vi "attachBall.vi"(0 "object in":refnum<class "KickToSkill.lvclass">, 1 "Dest":dbl[](array[numeric]), 2 "robotPos":dbl[](array[numeric]), 3 "Dist":dbl, 5 "error in (no error)":errorcluster) -> (14 "object out":refnum<class "KickToSkill.lvclass">, 15 "DestArray":dbl[](array[numeric]), 19 "error out":errorcluster)   [LabVIEW 2024, in "KickToSkill.lvclass"]
uses:
  KickToSkill.lvclass
  <vilib>/Analysis/coordinate.llb/2D Cartesian Coordinate Rotation (Scalar).vi
  <vilib>/Analysis/NI_AALPro.lvlib
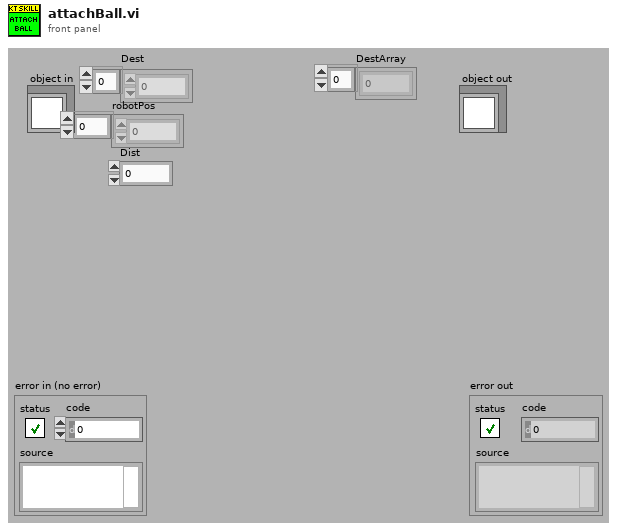
[diagram p1: front panel]
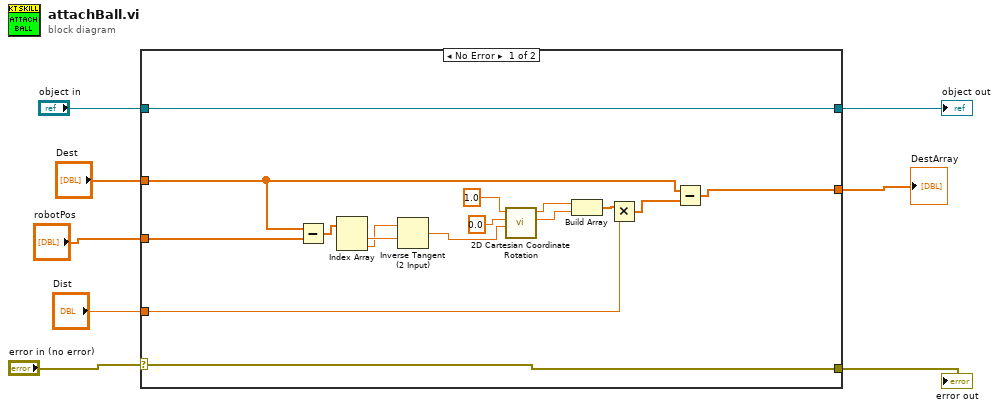
[diagram p0: block diagram]
diagram:
  n1 = case shown="No Error" "error in (no error)" {
    selector: "error in (no error)" -> [w23 w27]
    tunnel: [w23 w27] -> w7
    tunnel: [w24 w26] -> w5
    tunnel: "object in" -> [w24 w26]
    tunnel: [w15 w25] -> w4
    tunnel: "Dest" -> [w12 w25]
    tunnel: "Dist" -> [w14 _]
    tunnel: "robotPos" -> [w13 _]
    frame No Error {
      n2 = Subtract(x=w12, y=w13) -> (x-y=w11:dbl[])
      n3 = Index Array(array=w11) -> (element #1=w10:dbl, element #2=w9:dbl)  [unwired: 2 in]
      n4 = Inverse Tangent (2 Input)(1:w10, 2:w9) -> (0:w16:dbl)
      n5 = call-poly <vilib>:"2D Cartesian Coordinate Rotation.vi"("theta"=w16, "y"=0.0, "x"=1.0) -> ("y out"=w19:dbl, "x out"=w20:dbl)  [unwired: 6 in, 1 out]
      n6 = Build Array(w20, w19) -> (w18:dbl[])
      n7 = Multiply(x=w18, y=w14) -> (x*y=w17:dbl[])
      n8 = Subtract(x=w12, y=w17) -> (x-y=w15:dbl[])
    }
    frame Error {
    }
  }
  "error out" <- w7
  "object out" <- w5
  "DestArray" <- w4
